vi "Write VPA Error Log File.vi"(4 "Write File":bool=TRUE, 5 "Write Mode":bool, 6 "Initialize":bool, 7 "Error Out Mode":T1(ring), 8 "Error In":errorcluster, 10 "Test Mode":T2(ring), 11 "Log File Name":string="VPA Error.log") -> (0 "Error Out":errorcluster, 1 "Last Err":bool, 2 "Logged":bool, 3 "LineOut":string)   [LabVIEW 2013]
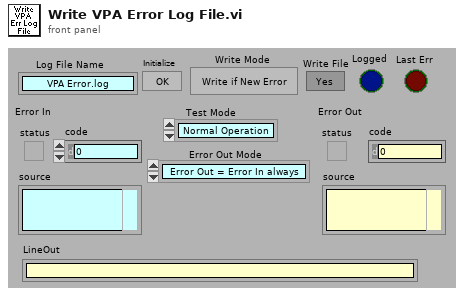
[diagram p1: front panel]
types:
  T1 = enum16{"Error Out = Error In always", "Always Cleared", "Error Out = Error In if Logged"}
  T2 = enum16{"Normal Operation", "Test - No Error", "Test - Error 1", "Test - Error 2"}
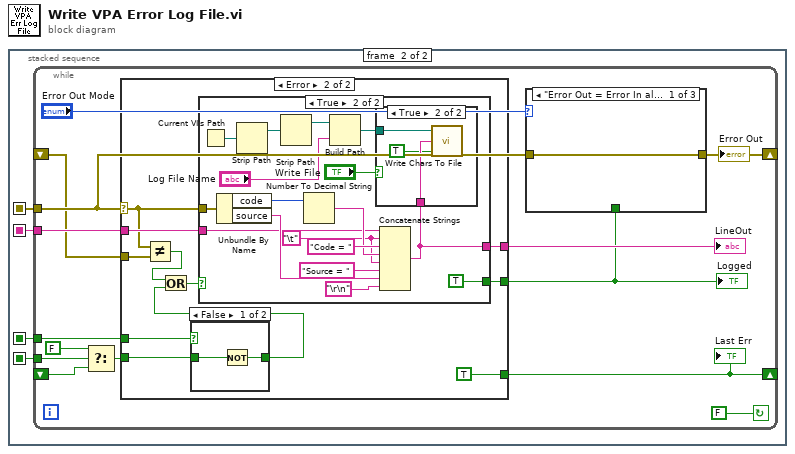
[diagram p0: block diagram]
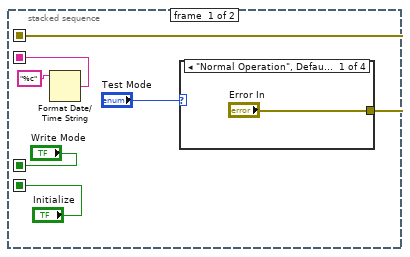
[diagram p2: hidden frame]
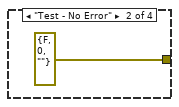
[diagram p3: hidden frame]
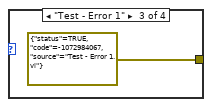
[diagram p4: hidden frame]
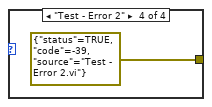
[diagram p5: hidden frame]
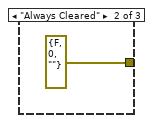
[diagram p6: hidden frame]
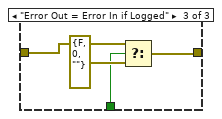
[diagram p7: hidden frame]
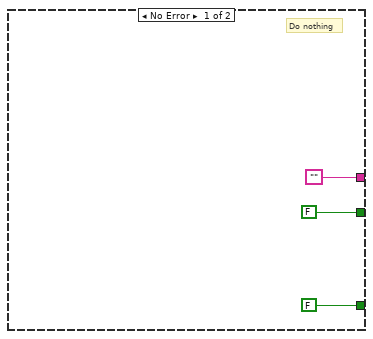
[diagram p8: hidden frame]
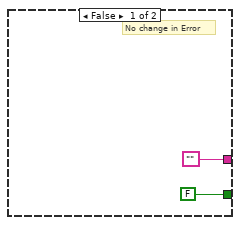
[diagram p9: hidden frame]
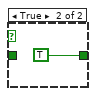
[diagram p11: hidden frame]
diagram:
  n1 = stacked-sequence {
    seq-local: [w3 _] -> [_ w14]
    seq-local: ["Write Mode" _] -> [_ w13]
    seq-local: ["Initialize" _] -> [_ w12]
    seq-local: [w1 _] -> [_ w11]
    frame #0 {
      n2 = Format Date/Time String(time format string (%c)="%c") -> (date/time string=w1:string)  [unwired: 2 in]
      n3 = case shown="\"Normal Operation\", Default" "Test Mode" {
        tunnel: ["Error In" errorcluster {"status"=FALSE, "code"=0, "source"=""} ("Error In") errorcluster {"status"=TRUE, "code"=-1072984067, "source"="Test - Error 1.vi"} ("Error In") errorcluster {"status"=TRUE, "code"=-39, "source"="Test - Error 2.vi"} ("Error In")] -> w3
        frame "Normal Operation", Default {
        }
        frame "Test - No Error" {
        }
        frame "Test - Error 1" {
        }
        frame "Test - Error 2" {
        }
      }
    }
    frame #1 {
      n4 = while {
        tunnel: w14 -> [w18]
        shift-right: [w20] -> _
        shift-left: _ -> [w25]
        tunnel: w13 -> [w27]
        tunnel: w12 -> [w26]
        tunnel: w11 -> [w22]
        shift-right: [w16] -> _
        shift-left: _ -> [w15]
        stop <- FALSE continue-if-true
        n5 = Select(t=FALSE, s=w26, f=w25) -> (s? t:f=w24:bool)
        n6 = case shown="Error" w18 {
          selector: w18 -> [_ w40]
          tunnel: w24 -> [_ w46]
          tunnel: [FALSE TRUE] -> w20
          tunnel: w27 -> [_ w47]
          tunnel: w22 -> [_ w45]
          tunnel: [FALSE w43] -> w17
          tunnel: ["" w42] -> w21
          tunnel: w15 -> [_ w39]
          frame No Error {
            # "Do nothing"
          }
          frame Error {
            n7 = Not Equal?(x=w40, y=w39) -> (x != y?=w38:bool)
            n8 = case shown="False" w47 {
              tunnel: w46 -> [w72 _]
              tunnel: [w71 TRUE] -> w44
              frame False {
                n9 = Not(x=w72) -> (.not. x?=w71:bool)
              }
              frame True {
              }
            }
            n10 = Or(x=w38, y=w44) -> (x .or. y?=w41:bool)
            n11 = case shown="True" w41 {
              tunnel: w40 -> [_ w62]
              tunnel: w45 -> [_ w53]
              tunnel: [FALSE TRUE] -> w43
              tunnel: ["" w51] -> w42
              frame False {
                # "No change in Error"
              }
              frame True {
                w57 = "\t"
                n12 = Current VI's Path() -> (path=w64:path)
                n13 = Unbundle By Name(w62) -> ("code"=w60:i32, "source"=w54:string)
                n14 = Strip Path(path=w64) -> (stripped path=w65:path)  [unwired: 1 out]
                n15 = Strip Path(path=w65) -> (stripped path=w66:path)  [unwired: 1 out]
                n16 = Number To Decimal String(number=w60) -> (decimal integer string=w58:string)  [unwired: 1 in]
                n17 = Build Path(base path=w66, name or relative path="Log File Name") -> (appended path=w63:path)
                n18 = Concatenate Strings(w53, w57, "Code = " ("string"), w58, w57, "Source = " ("string"), w54, "\r\n") -> (w51:string)
                n19 = case shown="True" "Write File" {
                  tunnel: w63 -> [_ w70]
                  tunnel: w51 -> [_ w69]
                  frame False {
                  }
                  frame True {
                    n20 = call "Write Chars To File.vi"("append to file? (new file:F)"=TRUE, "character string"=w69, "file path (dialog if empty)"=w70) -> ()  [unwired: 2 in, 1 out]
                  }
                }
              }
            }
          }
        }
        "Logged" <- w17
        "LineOut" <- w21
        "Last Err" <- w20
        n21 = case shown="\"Error Out = Error In always\", Default" "Error Out Mode" {
          tunnel: [w29 errorcluster {"status"=FALSE, "code"=0, "source"=""} ("Error In") w33] -> w16
          tunnel: w18 -> [w29 _ w32]
          tunnel: w17 -> [_ _ w31]
          frame "Error Out = Error In always", Default {
          }
          frame "Always Cleared" {
          }
          frame "Error Out = Error In if Logged" {
            n22 = Select(t=w32, s=w31, f=errorcluster {"status"=FALSE, "code"=0, "source"=""} ("Error In")) -> (s? t:f=w33:errorcluster)
          }
        }
        "Error Out" <- w16
      }
    }
  }
